vi "ControlMethod.vi"() -> ()   [LabVIEW 2014]
uses:
  Libraries/Contact Data/Contact.ctl
  Libraries/Contact Data/Position.ctl
  Libraries/Contact Data/Controls.ctl
  Libraries/Contact Data/DestinationCluster.ctl
  Libraries/Contact Data/DesinationControls.ctl
  Libraries/Contact Data/PathData.ctl
  PathFinder/Controls/ShortestPath.ctl
  Libraries/Map Data Folder/CursorList.ctl
  Libraries/Contact Data/Contact Data.lvlib
  Libraries/Map Data Folder/Map Data.lvlib
panel:
  in  "Numeric":i32
  in  "input cluster":T1={"ID"=0, "UUID"="", "Name"="", "Iteration"=0, "Posit Array"=[], "Controls"={"throttle"=0.0, "brake"=0.0, "horn"=0.0, "wait"=0.5}, "DestArray"=[], "SetSpeed"=0.0, "Speed"=0.0, "PathData"={"Path Found?"=FALSE, "Same Line +Dir?"=FALSE, "Path"=[], "Distance to Dest"=0.0}}
  in  "Divide by":dbl=100.0
  in  "Max throttle":dbl=0.8 format="%#_13g"
  out "PID output":dbl[](array[numeric])=[100.0, 100.0] format="%.2f"
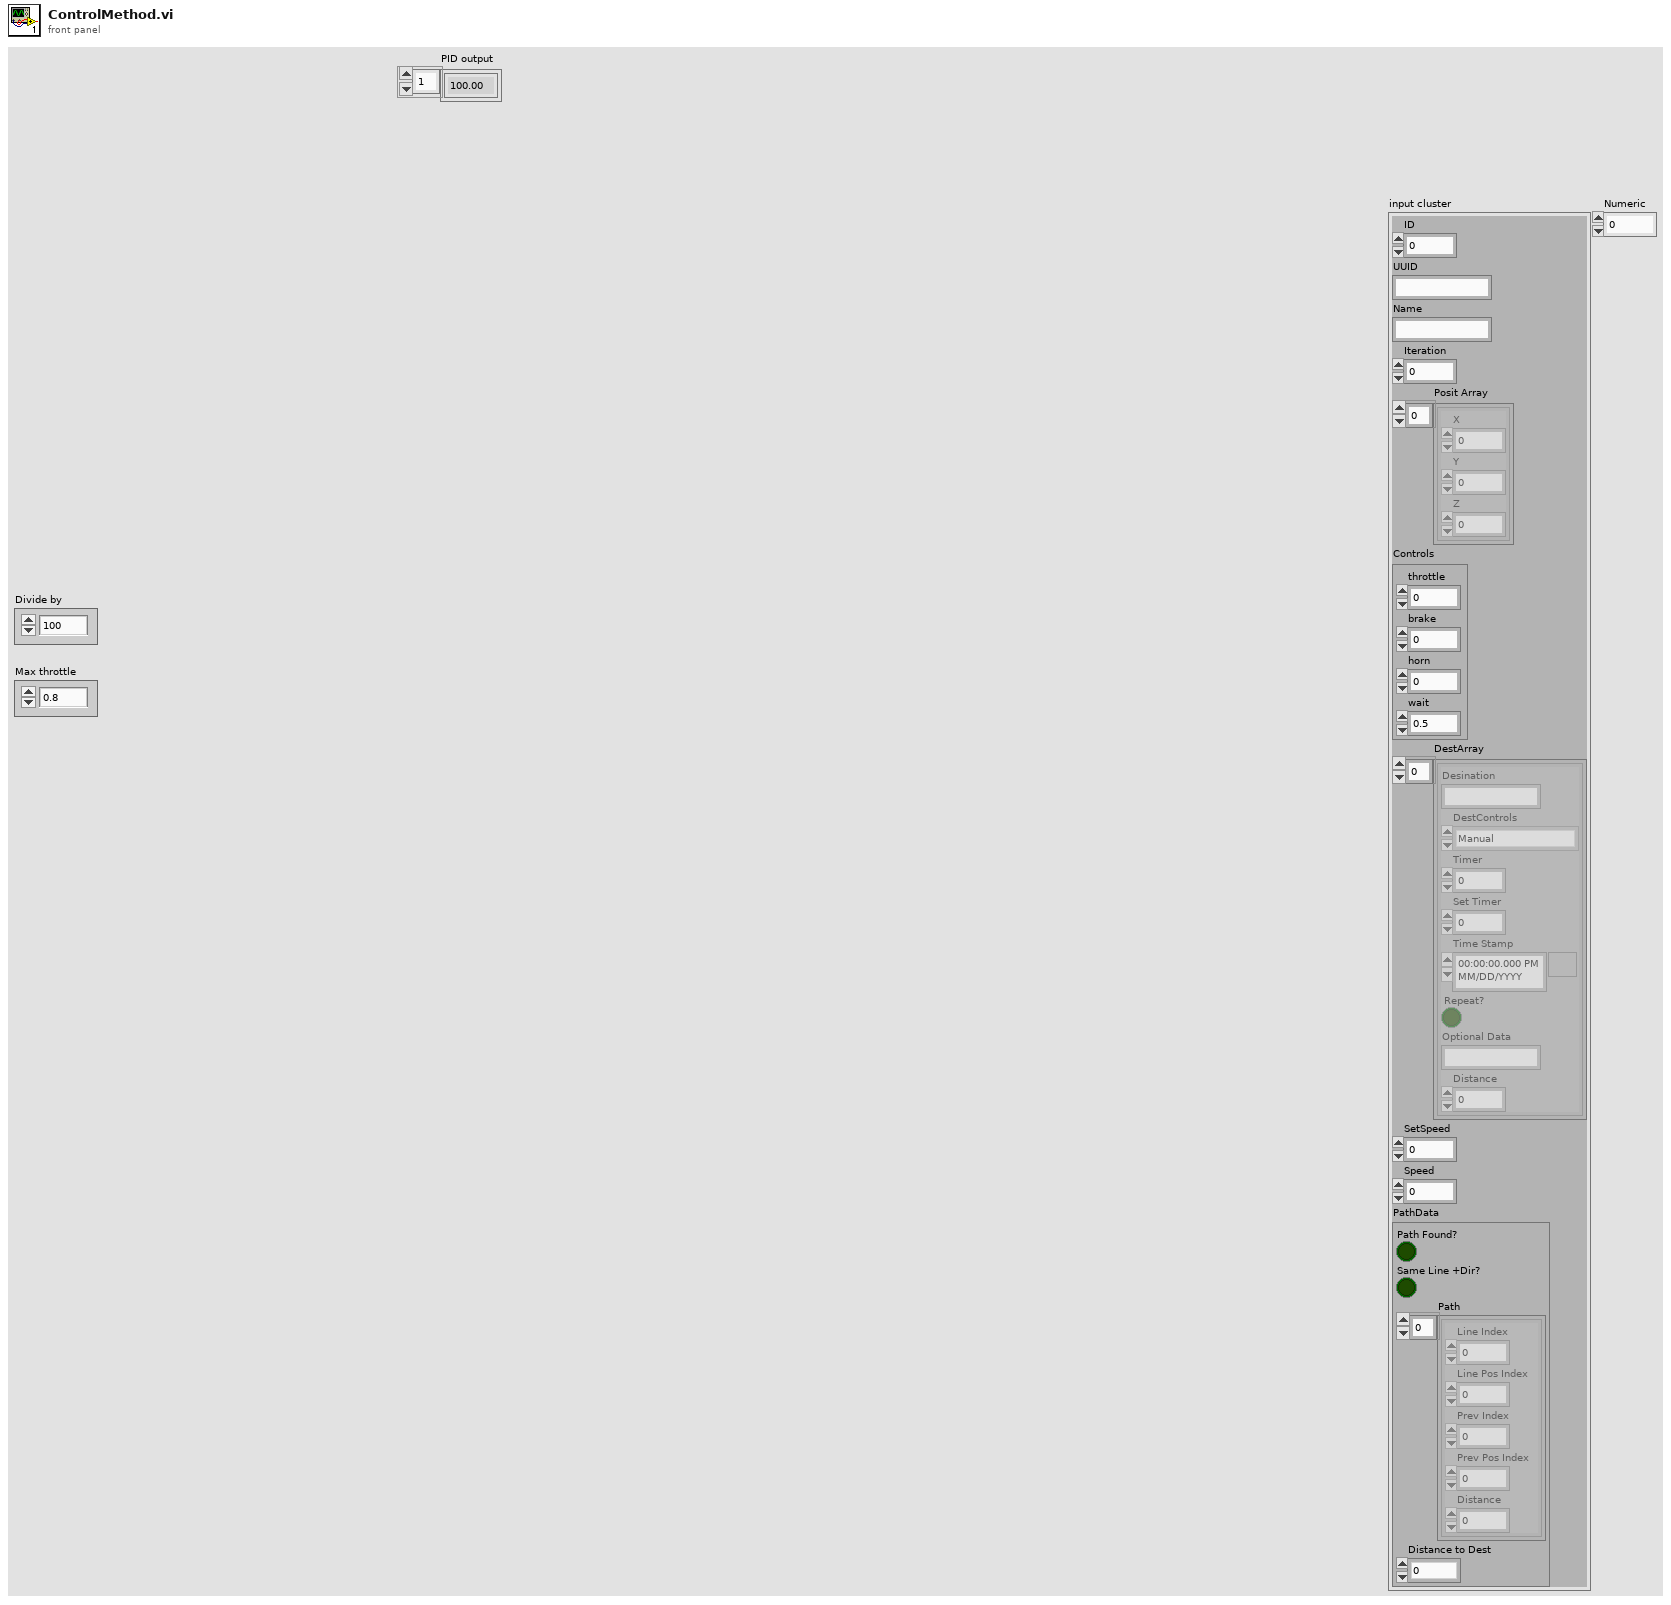
[diagram p1: front panel]
types:
  T1 = typedef "Contact Data.lvlib/Contact.ctl" = cluster{"ID":u32, "UUID":string, "Name":string, "Iteration":i32, "Posit Array":T2[], "Controls":T3, "DestArray":T4[], "SetSpeed":dbl, "Speed":dbl, "PathData":T6}
  T2 = typedef "Contact Data.lvlib/Position.ctl" = cluster{"X":dbl, "Y":dbl, "Z":dbl}
  T3 = typedef "Contact Data.lvlib/Controls.ctl" = cluster{"throttle":dbl, "brake":dbl, "horn":dbl, "wait":dbl}
  T4 = typedef "Contact Data.lvlib/DestinationCluster.ctl" = cluster{"Desination":string, "DestControls":T5, "Timer":u32, "Set Timer":u32, "Time Stamp":timestamp, "Repeat?":bool, "Optional Data":string, "Distance":dbl}
  T5 = typedef "Contact Data.lvlib/DesinationControls.ctl" = enum16{"Tracker", "Manual", "Stop", "Station DateTime", "Station Timer", "Maintain"}
  T6 = typedef "Contact Data.lvlib/PathData.ctl" = cluster{"Path Found?":bool, "Same Line +Dir?":bool, "Path":T7[], "Distance to Dest":dbl}
  T7 = typedef "ShortestPath.ctl" = cluster{"Line Index":i32, "Line Pos Index ":i32, "Prev Index ":i32, "Prev Pos Index":i32, "Distance":dbl}
  T8 = cluster{"In Area(1)":dbl, "Entering Station(2)":dbl, "Final Approach(3)":dbl, "At Dest(4)":dbl}
  T9 = typedef "Map Data.lvlib/CursorList.ctl" = cluster{"Name":string, "Color":u32, "Style":u8, "Point Style":u8, "Name Visible":bool, "Allow Drag":bool, "Cursor Mode":u32, "Plot":i32, "Index":i32, "Position":cluster{"X":dbl, "Y":dbl}, "X Scale":u32, "Y Scale":u32, "Watch Plots":i32[], "Watch All Plots":bool, "Plot Area":i32, "Label Offset":cluster{"X":dbl, "Y":dbl}}[]
  T10 = cluster{"In Area(1)":bool, "Entering Station(2)":bool, "Final Approach(3)":bool, "At Dest(4)":bool}
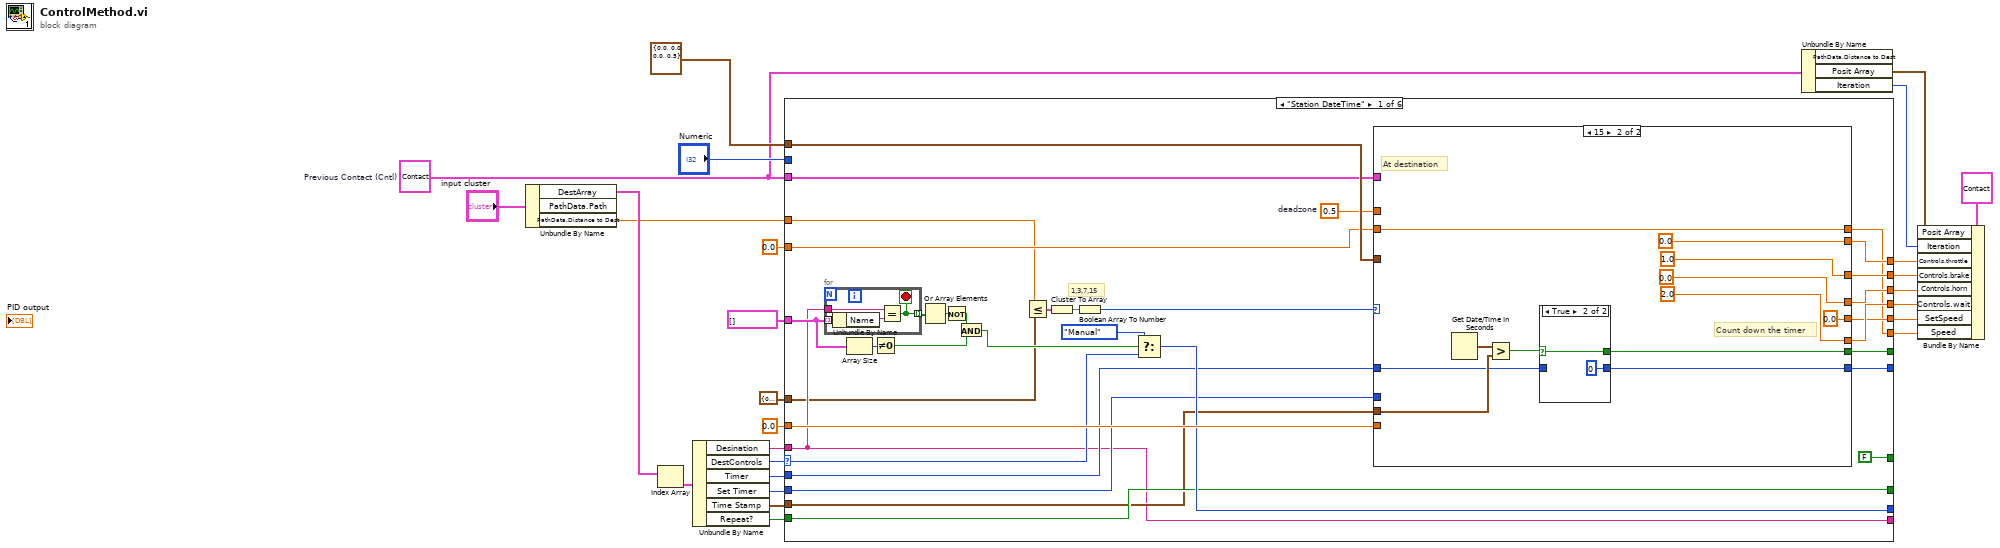
[diagram p0: block diagram]
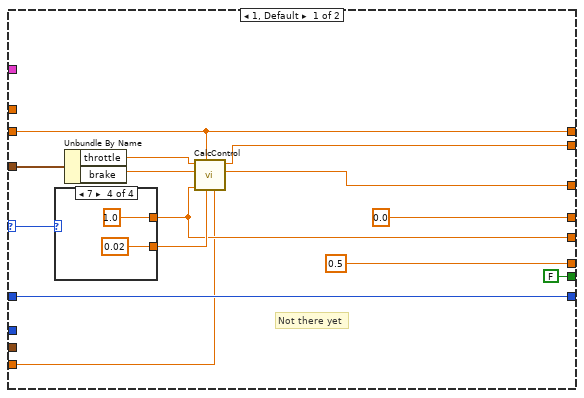
[diagram p2: hidden frame]
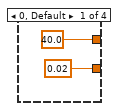
[diagram p3: hidden frame]
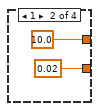
[diagram p4: hidden frame]
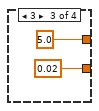
[diagram p5: hidden frame]
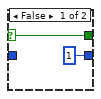
[diagram p6: hidden frame]
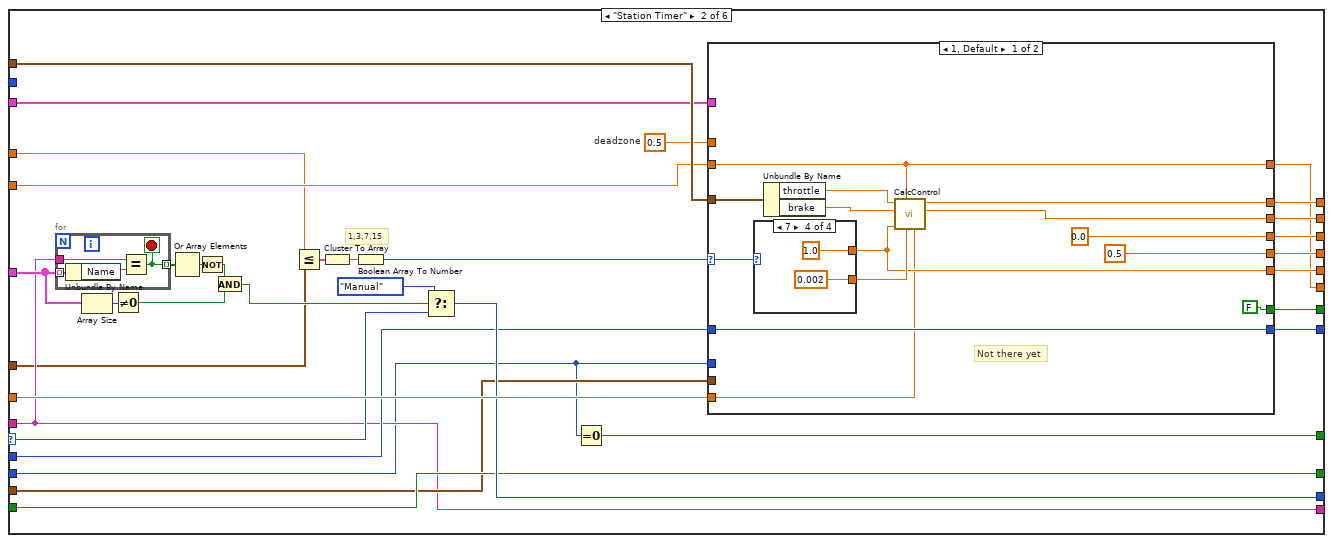
[diagram p7: hidden frame]
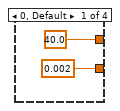
[diagram p8: hidden frame]
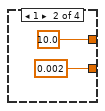
[diagram p9: hidden frame]
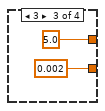
[diagram p10: hidden frame]
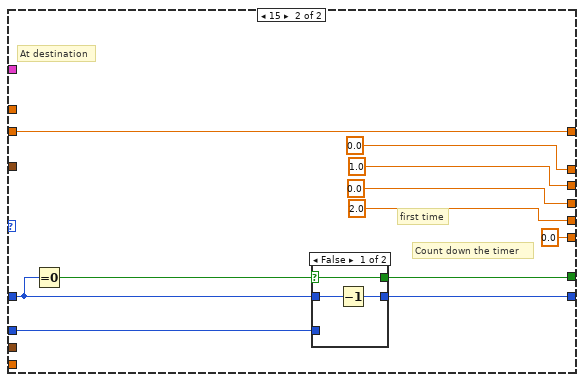
[diagram p11: hidden frame]
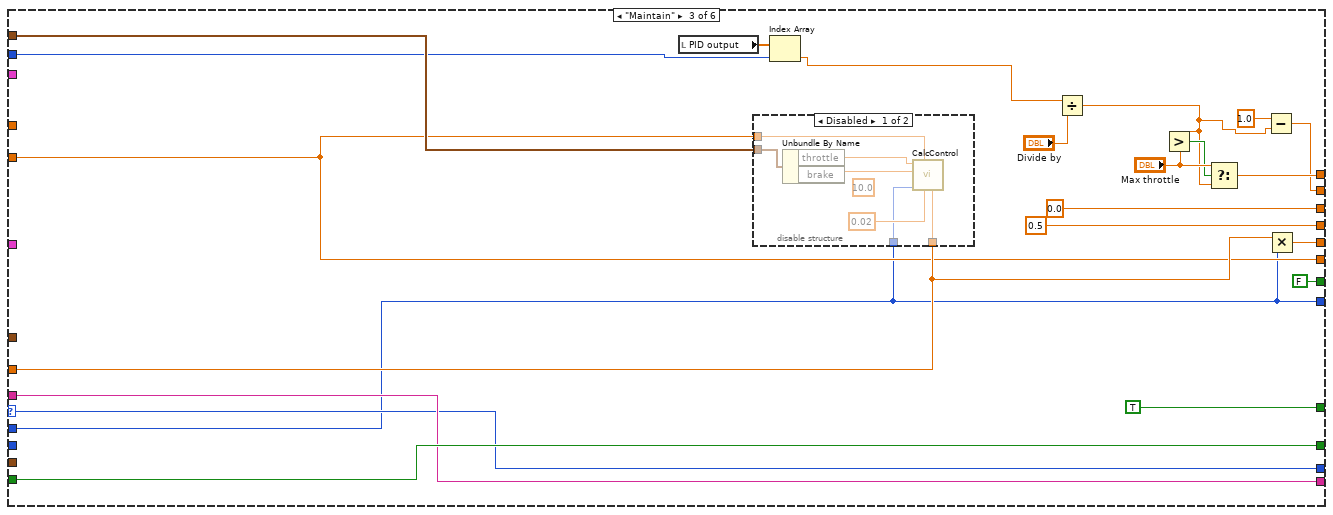
[diagram p13: hidden frame]
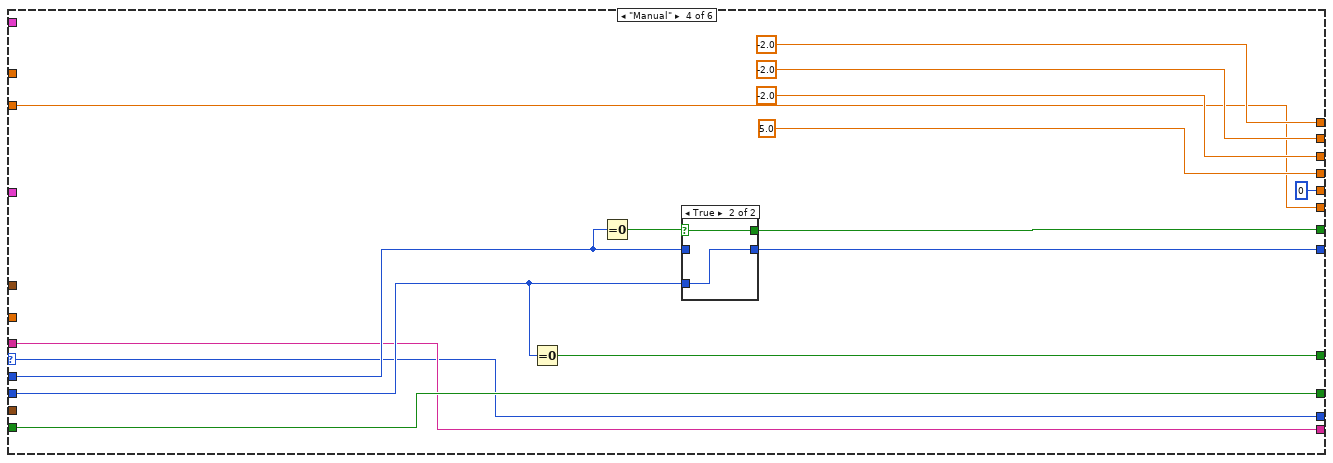
[diagram p15: hidden frame]
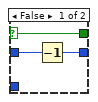
[diagram p16: hidden frame]
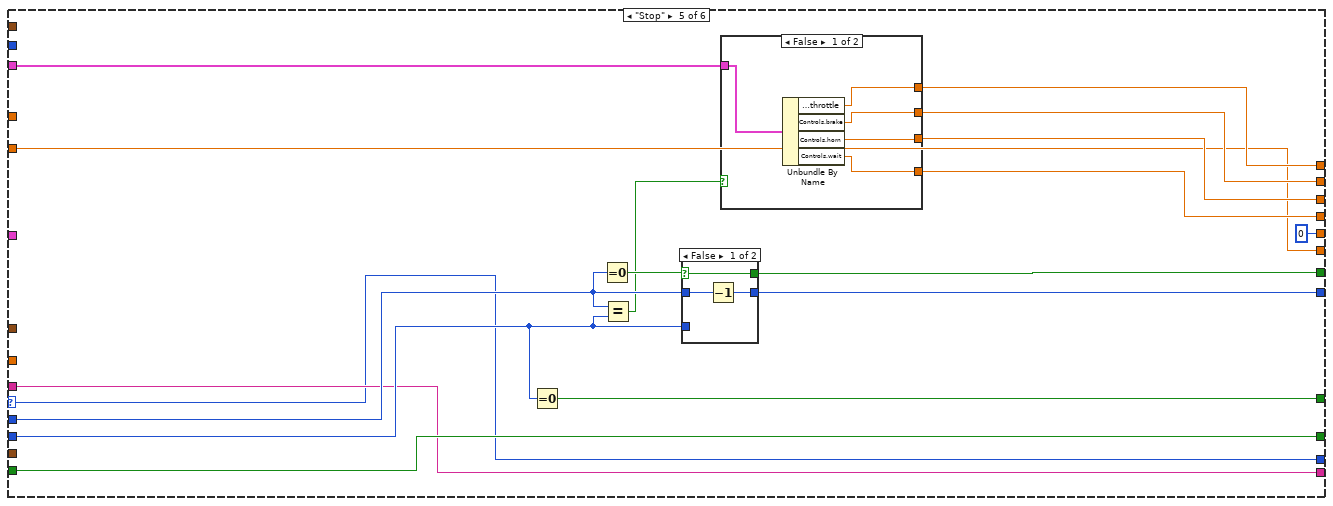
[diagram p17: hidden frame]
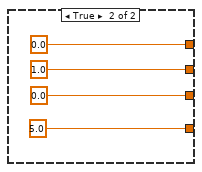
[diagram p18: hidden frame]
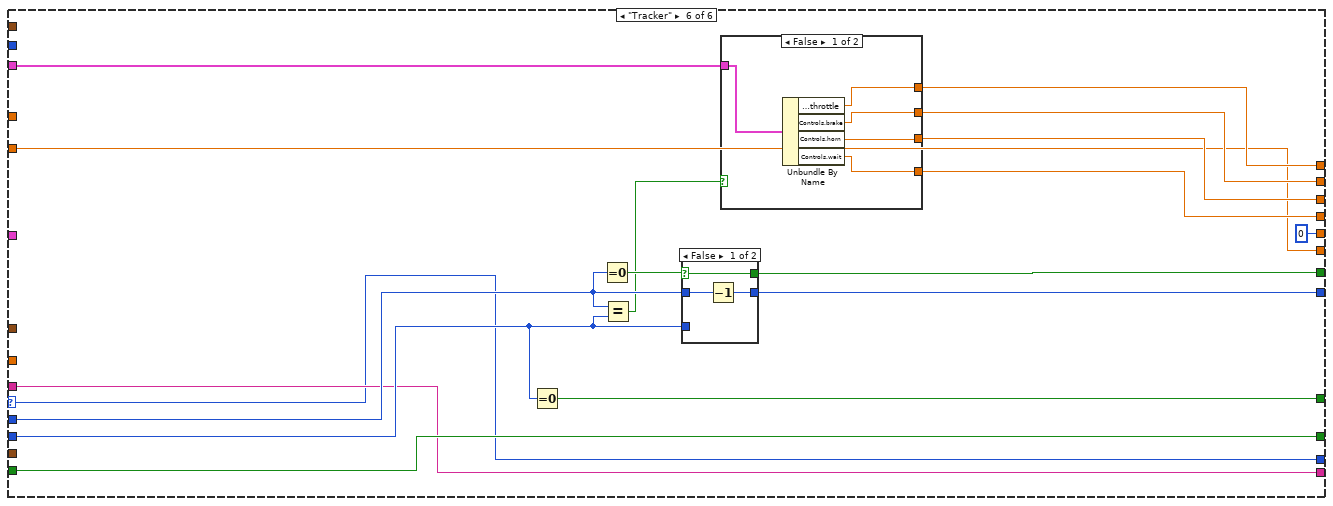
[diagram p20: hidden frame]
diagram:
  w1 = T1 {"ID"=0, "UUID"="", "Name"="", "Iteration"=0, "Posit Array"=[], "Controls"={"throttle"=0.0, "brake"=0.0, "horn"=0.0, "wait"=0.5}, "DestArray"=[], "SetSpeed"=0.0, "Speed"=0.0, "PathData"={"Path Found?"=FALSE, "Same Line +Dir?"=FALSE, "Path"=[], "Distance to Dest"=0.0}}  # Previous Contact (Cntl)
  n1 = Unbundle By Name("input cluster") -> ("DestArray"=w25:T4[], "PathData.Distance to Dest"=w6:dbl)  [unwired: 1 out]
  n2 = Index Array(array=w25) -> (element=w23:T4)  [unwired: 1 in]
  n3 = Unbundle By Name(w23) -> ("Desination"=w26:string, "DestControls"=w18:T5, "Timer"=w19:u32, "Set Timer"=w20:u32, "Time Stamp"=w21:timestamp, "Repeat?"=w22:bool)
  n4 = case shown="\"Station DateTime\"" w18 {
    selector: w18 -> [w44 w121 w194 w210 w231 w262]
    tunnel: T3 {"throttle"=0.0, "brake"=0.0, "horn"=0.0, "wait"=0.5} ("Controls") -> [w60 w136 w200 _ _ _]
    tunnel: w26 -> [w39 w117 w195 w212 w234 w265]
    tunnel: [w58 w134 FALSE w222 w244 w275] -> _
    tunnel: [w57 w133 w183 w221 w243 w274] -> _
    tunnel: 0.0 -> [w56 w132 w184 w209 w229 w260]
    tunnel: [w55 w131 0.5 ("Controls.brake") 5.0 ("Controls.brake") w242 w273] -> w14
    tunnel: [w54 w130 w189 -2.0 ("Controls.brake") w241 w272] -> w11
    tunnel: [w53 w129 w182 -2.0 ("Controls.brake") w240 w271] -> w12
    tunnel: [w52 w128 0.0 ("Controls.brake") -2.0 ("Controls.brake") w239 w270] -> w13
    tunnel: [FALSE w103 TRUE w216 w238 w269] -> _
    tunnel: w1 -> [w37 w115 _ _ w230 w261]
    tunnel: [w43 w120 w196 w215 w237 w268] -> _
    tunnel: 0.0 ("Multiplier") -> [w49 w126 w185 _ _ _]
    tunnel: [w48 w125 w194 w210 w231 w262] -> _
    tunnel: T9 [] ("Cursor List") -> [w45 w122 _ _ _ _]
    tunnel: [w39 w117 w195 w212 w234 w265] -> _
    tunnel: w19 -> [w40 w118 w183 w213 w235 w266]
    tunnel: w20 -> [w41 w104 _ w214 w236 w267]
    tunnel: w21 -> [w42 w119 _ _ _ _]
    tunnel: w22 -> [w43 w120 w196 w215 w237 w268]
    tunnel: [w36 w114 w186 u32 0 ("Timer") u32 0 ("Timer") u32 0 ("Timer")] -> w15
    tunnel: [w35 w113 w184 w209 w229 w260] -> w16
    tunnel: "Numeric" -> [_ _ w187 _ _ _]
    tunnel: w6 -> [w31 w109 _ _ _ _]
    tunnel: T8 {"In Area(1)"=0.0, "Entering Station(2)"=0.0, "Final Approach(3)"=0.0, "At Dest(4)"=0.0} -> [w30 w108 _ _ _ _]
    frame "Station DateTime" {
      w38 = 0.5  # deadzone
      # "1,3,7,15"
      n5 = for {
        tunnel: w39 -> [w100]
        tunnel: w45 -> [w101] mode=indexing
        tunnel: [w99] -> w50 mode=indexing
        stop <- w99 stop-if-true
        n6 = Unbundle By Name(w101) -> ("Name"=w102:string)
        n7 = Equal?(x=w100, y=w102) -> (x = y?=w99:bool)
      }
      n8 = Array Size(array=w45) -> (size(s)=w46:i32)
      n9 = Not Equal To 0?(x=w46) -> (x != 0?=w33:bool)
      n10 = Or Array Elements(Boolean array=w50) -> (logical OR=w47:bool)
      n11 = Not(x=w47) -> (.not. x?=w34:bool)
      n12 = And(x=w34, y=w33) -> (x .and. y?=w32:bool)
      n13 = Less Or Equal?(x=w31, y=w30) -> (x <= y?=w29:T10)
      n14 = Cluster To Array(cluster=w29) -> (array=w28:bool[])
      n15 = Boolean Array To Number(Boolean array=w28) -> (number=w27:u32)
      n16 = Select(t=DesinationControls."Manual", s=w32, f=w44) -> (s? t:f=w48:T5)
      n17 = case shown="15" w27 {
        selector: w27 -> [w61 _]
        tunnel: w37 -> [_ _]
        tunnel: w40 -> [w73 w85]
        tunnel: [FALSE w86] -> w58
        tunnel: [w73 w88] -> w57
        tunnel: w41 -> [_ _]
        tunnel: w56 -> [w62 w83]
        tunnel: w38 -> [_ _]
        tunnel: w60 -> [w64 _]
        tunnel: [w65 0.0 ("Controls.brake")] -> w54
        tunnel: [0.5 ("Controls.brake") 2.0 ("Controls.brake")] -> w55
        tunnel: [w66 1.0 ("Controls.brake")] -> w53
        tunnel: [0.0 ("Controls.brake") 0.0 ("Controls.brake")] -> w52
        tunnel: w42 -> [_ w89]
        tunnel: w49 -> [w63 _]
        tunnel: [w67 0.0] -> w36
        tunnel: [w62 w83] -> w35
        frame 1, Default {
          # "Not there yet"
          n18 = case shown="7" w61 {
            tunnel: [0.02 ("Change Throttle") 0.02 ("Change Throttle") 0.02 ("Change Throttle") 0.02 ("Change Throttle")] -> w70
            tunnel: [40.0 10.0 5.0 1.0] -> w67
            frame 0, Default {
            }
            frame 1 {
            }
            frame 3 {
            }
            frame 7 {
            }
          }
          n19 = Unbundle By Name(w64) -> ("throttle"=w72:dbl, "brake"=w71:dbl)
          n20 = call "CalcControl.vi"("Multiplier"=w63, "Change Throttle"=w70, "Current Speed"=w62, "Set Speed"=w67, "Current Brake"=w71, "Current Throttle"=w72) -> ("New Brake"=w66:dbl, "New Throttle"=w65:dbl)  [unwired: 3 in, 1 out]
        }
        frame 15 {
          # "At destination"
          # "Count down the timer"
          n21 = Get Date/Time In Seconds() -> (seconds since 1Jan1904=w90:timestamp)
          n22 = Greater?(x=w90, y=w89) -> (0:w87:bool)
          n23 = case shown="True" w87 {
            selector: w87 -> [w96 w97]
            tunnel: w85 -> [_ _]
            tunnel: [u32 1 ("Timer") u32 0 ("Timer")] -> w88
            tunnel: [w96 w97] -> w86
            frame False {
            }
            frame True {
            }
          }
        }
      }
    }
    frame "Station Timer" {
      w116 = 0.5  # deadzone
      # "1,3,7,15"
      n24 = for {
        tunnel: w117 -> [w176]
        tunnel: w122 -> [w177] mode=indexing
        tunnel: [w175] -> w127 mode=indexing
        stop <- w175 stop-if-true
        n25 = Unbundle By Name(w177) -> ("Name"=w178:string)
        n26 = Equal?(x=w176, y=w178) -> (x = y?=w175:bool)
      }
      n27 = Array Size(array=w122) -> (size(s)=w123:i32)
      n28 = Not Equal To 0?(x=w123) -> (x != 0?=w111:bool)
      n29 = Or Array Elements(Boolean array=w127) -> (logical OR=w124:bool)
      n30 = Not(x=w124) -> (.not. x?=w112:bool)
      n31 = And(x=w112, y=w111) -> (x .and. y?=w110:bool)
      n32 = Less Or Equal?(x=w109, y=w108) -> (x <= y?=w107:T10)
      n33 = Cluster To Array(cluster=w107) -> (array=w106:bool[])
      n34 = Boolean Array To Number(Boolean array=w106) -> (number=w105:u32)
      n35 = Select(t=DesinationControls."Manual", s=w110, f=w121) -> (s? t:f=w125:T5)
      n36 = Equal To 0?(x=w104) -> (x = 0?=w103:bool)
      n37 = case shown="1, Default" w105 {
        selector: w105 -> [w137 _]
        tunnel: w115 -> [_ _]
        tunnel: w118 -> [w149 w160]
        tunnel: [FALSE w161] -> w134
        tunnel: [w149 w162] -> w133
        tunnel: w104 -> [_ w159]
        tunnel: w132 -> [w138 w164]
        tunnel: w116 -> [_ _]
        tunnel: w136 -> [w140 _]
        tunnel: [w141 0.0 ("Controls.brake")] -> w130
        tunnel: [0.5 ("Controls.brake") 2.0 ("Controls.brake")] -> w131
        tunnel: [w142 1.0 ("Controls.brake")] -> w129
        tunnel: [0.0 ("Controls.brake") 0.0 ("Controls.brake")] -> w128
        tunnel: w119 -> [_ _]
        tunnel: w126 -> [w139 _]
        tunnel: [w143 0.0] -> w114
        tunnel: [w138 w164] -> w113
        frame 1, Default {
          # "Not there yet"
          n38 = case shown="7" w137 {
            tunnel: [0.002 ("Change Throttle") 0.002 ("Change Throttle") 0.002 ("Change Throttle") 0.002 ("Change Throttle")] -> w146
            tunnel: [40.0 10.0 5.0 1.0] -> w143
            frame 0, Default {
            }
            frame 1 {
            }
            frame 3 {
            }
            frame 7 {
            }
          }
          n39 = Unbundle By Name(w140) -> ("throttle"=w148:dbl, "brake"=w147:dbl)
          n40 = call "CalcControl.vi"("Multiplier"=w139, "Change Throttle"=w146, "Current Speed"=w138, "Set Speed"=w143, "Current Brake"=w147, "Current Throttle"=w148) -> ("New Brake"=w142:dbl, "New Throttle"=w141:dbl)  [unwired: 3 in, 1 out]
        }
        frame 15 {
          # "first time"
          # "At destination"
          # "Count down the timer"
          n41 = Equal To 0?(x=w160) -> (x = 0?=w163:bool)
          n42 = case shown="False" w163 {
            selector: w163 -> [w172 w174]
            tunnel: w160 -> [w171 _]
            tunnel: [w170 w173] -> w162
            tunnel: [w172 w174] -> w161
            tunnel: w159 -> [_ w173]
            frame False {
              n43 = Decrement(x=w171) -> (x-1=w170:u32)
            }
            frame True {
            }
          }
        }
      }
    }
    frame "Maintain" {
      n44 = local read "PID output"() -> (w188:dbl[])
      n45 = disable-structure shown="Disabled" {
        disable-tunnel: w200 -> [w207 _]
        disable-tunnel: w185 -> [w206 _]
        disable-tunnel: w184 -> [w203 _]
        disable-tunnel: w183 -> [w202 _]
        frame Disabled {
          (unwired) 10.0
          n46 = Unbundle By Name(w207) -> ("throttle"=w205:dbl, "brake"=w201:dbl)
          n47 = call "CalcControl.vi"("Multiplier"=w206, "Change Throttle"=0.02, "Current Speed"=w203, "Set Speed"=w202, "Current Brake"=w201, "Current Throttle"=w205) -> ()  [unwired: 3 in, 3 out]
        }
        frame Enabled {
        }
      }
      n48 = Index Array(array=w188, index=w187) -> (element=w181:dbl)
      n49 = Divide(x=w181, y="Divide by") -> (x/y=w179:dbl)
      n50 = Greater?(x=w179, y="Max throttle") -> (0:w190:bool)
      n51 = Select(t="Max throttle", s=w190, f=w179) -> (s? t:f=w189:dbl)
      n52 = Subtract(x=1.0, y=w179) -> (x-y=w182:dbl)
      n53 = Multiply(x=w185, y=w183) -> (x*y=w186:dbl)
    }
    frame "Manual" {
      n54 = Equal To 0?(x=w214) -> (x = 0?=w216:bool)
      n55 = Equal To 0?(x=w213) -> (x = 0?=w211:bool)
      n56 = case shown="True" w211 {
        selector: w211 -> [w225 w227]
        tunnel: w213 -> [w224 _]
        tunnel: [w223 w226] -> w221
        tunnel: [w225 w227] -> w222
        tunnel: w214 -> [_ w226]
        frame False {
          n57 = Decrement(x=w224) -> (x-1=w223:u32)
        }
        frame True {
        }
      }
    }
    frame "Stop" {
      n58 = Equal To 0?(x=w236) -> (x = 0?=w238:bool)
      n59 = Equal To 0?(x=w235) -> (x = 0?=w233:bool)
      n60 = Equal?(x=w235, y=w236) -> (x = y?=w232:bool)
      n61 = case shown="False" w233 {
        selector: w233 -> [w256 w258]
        tunnel: w235 -> [w255 _]
        tunnel: [w254 w257] -> w243
        tunnel: [w256 w258] -> w244
        tunnel: w236 -> [_ w257]
        frame False {
          n62 = Decrement(x=w255) -> (x-1=w254:u32)
        }
        frame True {
        }
      }
      n63 = case shown="False" w232 {
        tunnel: w230 -> [w249 _]
        tunnel: [w248 0.0 ("Controls.brake")] -> w241
        tunnel: [w247 1.0 ("Controls.brake")] -> w240
        tunnel: [w246 0.0 ("Controls.brake")] -> w239
        tunnel: [w245 5.0 ("Controls.brake")] -> w242
        frame False {
          n64 = Unbundle By Name(w249) -> ("Controls.throttle"=w248:dbl, "Controls.brake"=w247:dbl, "Controls.horn"=w246:dbl, "Controls.wait"=w245:dbl)
        }
        frame True {
        }
      }
    }
    frame "Tracker" {
      n65 = Equal To 0?(x=w267) -> (x = 0?=w269:bool)
      n66 = Equal To 0?(x=w266) -> (x = 0?=w264:bool)
      n67 = Equal?(x=w266, y=w267) -> (x = y?=w263:bool)
      n68 = case shown="False" w264 {
        selector: w264 -> [w287 w289]
        tunnel: w266 -> [w286 _]
        tunnel: [w285 w288] -> w274
        tunnel: [w287 w289] -> w275
        tunnel: w267 -> [_ w288]
        frame False {
          n69 = Decrement(x=w286) -> (x-1=w285:u32)
        }
        frame True {
        }
      }
      n70 = case shown="False" w263 {
        tunnel: w261 -> [w280 _]
        tunnel: [w279 -2.0 ("Controls.brake")] -> w272
        tunnel: [w278 -2.0 ("Controls.brake")] -> w271
        tunnel: [w277 -2.0 ("Controls.brake")] -> w270
        tunnel: [w276 0.5 ("Controls.brake")] -> w273
        frame False {
          n71 = Unbundle By Name(w280) -> ("Controls.throttle"=w279:dbl, "Controls.brake"=w278:dbl, "Controls.horn"=w277:dbl, "Controls.wait"=w276:dbl)
        }
        frame True {
        }
      }
    }
  }
  n72 = Unbundle By Name(w1) -> ("Posit Array"=w24:T2[], "Iteration"=w10:i32)  [unwired: 1 out]
  n73 = Bundle By Name(cluster=T1 {"ID"=0, "UUID"="", "Name"="", "Iteration"=0, "Posit Array"=[], "Controls"={"throttle"=0.0, "brake"=0.0, "horn"=0.0, "wait"=0.5}, "DestArray"=[], "SetSpeed"=0.0, "Speed"=0.0, "PathData"={"Path Found?"=FALSE, "Same Line +Dir?"=FALSE, "Path"=[], "Distance to Dest"=0.0}} ("input cluster"), "Posit Array"=w24, "Iteration"=w10, "Controls.throttle"=w11, "Controls.brake"=w12, "Controls.horn"=w13, "Controls.wait"=w14, "SetSpeed"=w15, "Speed"=w16) -> ()  [unwired: 1 out]
